vi "SysTime.vi"(5 "Function":enum16{"get_time", "set_time"}(ring), 6 "error in (no error)":errorcluster, 9 "SYSTEMTIME in":T1) -> (0 "error out":errorcluster, 3 "SYSTEMTIME out":T1)   [LabVIEW 2011]
doc: "This VI acts as a Win32 System Call wrapper. Embedded within the VI are \"Call Library\" functions which call various functions from the KERNEL32, GDI, and USER dynamically linked libraries (.DLL's) found in the Windows\\System directory.\n\nThe input is an Enumerated U16 which describes the type of system call to make, and which of the VI's input/output terminals to utilize. A generic \"error?\" boolean is output to indicate any errors with the function calls.\n\nList of Functions and Input/Output Terminals:\n---------------------------------------------------------------------------------------------------------------\n0) get_time: uses the \"SYSTEMTIME out\" terminal only. This call retrieves the system time according to the CPU and operating system. The output is a cluster of eight U16's (the same as the Win32 API description of the SYSTEMTIME structure).\n\n1) set_time: uses both the \"SYSTEMTIME\" and \"SYSTEMTIME out\" terminals. This call will set the system clock to the time and date indicated in the input structure (cluster)."
uses:
  KERNEL32.DLL
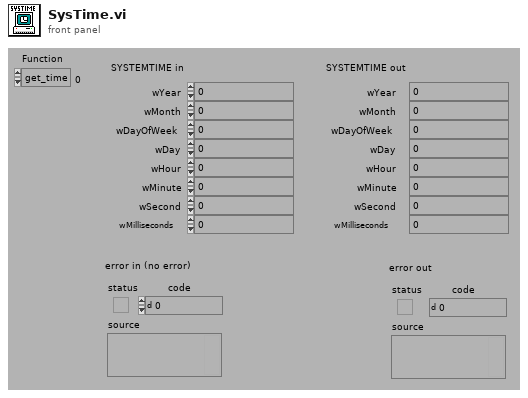
[diagram p1: front panel]
types:
  T1 = cluster{"wYear":u16, "wMonth":u16, "wDayOfWeek":u16, "wDay":u16, "wHour":u16, "wMinute":u16, "wSecond":u16, "wMilliseconds":u16}
  T2 = cluster{"SysTimeStruct[0]":u16, "SysTimeStruct[1]":u16, "SysTimeStruct[2]":u16, "SysTimeStruct[3]":u16, "SysTimeStruct[4]":u16, "SysTimeStruct[5]":u16, "SysTimeStruct[6]":u16, "SysTimeStruct[7]":u16}
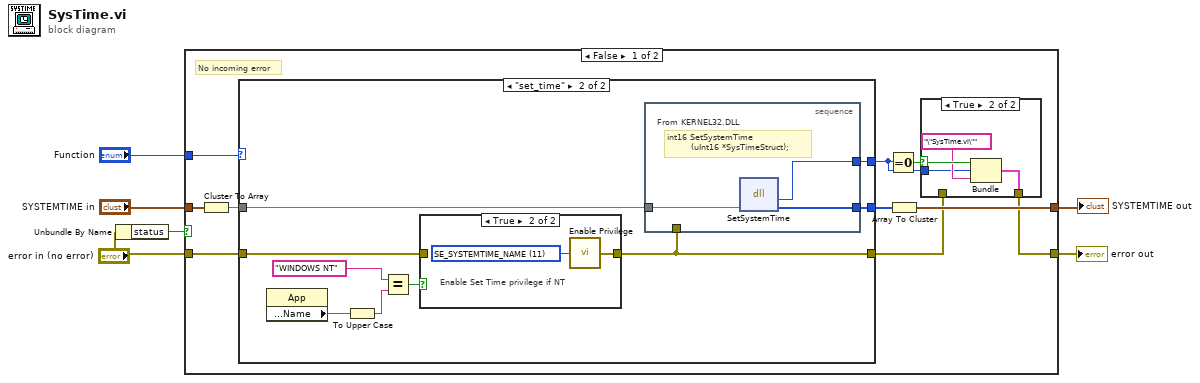
[diagram p0: block diagram]
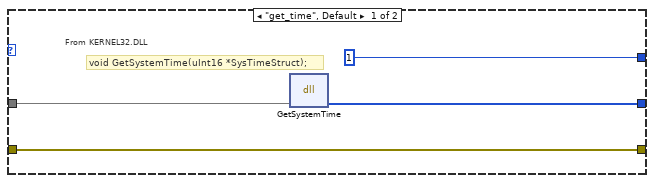
[diagram p3: hidden frame]
diagram:
  n1 = Unbundle By Name("error in (no error)") -> ("status"=w3:bool)
  n2 = case shown="False" w3 {
    tunnel: "SYSTEMTIME in" -> [w16 w41]
    tunnel: [w15 w41] -> w5
    tunnel: "Function" -> [w12 _]
    tunnel: [w10 w42] -> w1
    tunnel: "error in (no error)" -> [w8 w42]
    frame False {
      # "No incoming error"
      n3 = Cluster To Array(cluster=w16) -> (array=w13:u16[])
      n4 = case shown="\"set_time\"" w12 {
        tunnel: [w25 w33] -> w14
        tunnel: w13 -> [w24 w34]
        tunnel: [i16 1 w32] -> w9
        tunnel: w8 -> [w22 w27]
        tunnel: [w22 w26] -> w7
        frame "get_time", Default {
          # "void GetSystemTime(uInt16 *SysTimeStruct);"
          # "From KERNEL32.DLL"
          n5 = dll-call lib="KERNEL32.DLL" fn="GetSystemTime"("SysTimeStruct"=w24) -> ("SysTimeStruct"=w25:u16[])  [unwired: 4 in, 2 out]
        }
        frame "set_time" {
          n6 = property class="App"() -> ("Operating System:Name"=w29:string)  [unwired: 2 in, 2 out]
          n7 = To Upper Case(1:w29) -> (0:w31:string)
          n8 = Equal?(x="WINDOWS NT", y=w31) -> (x = y?=w28:bool)
          n9 = case shown="True" w28 {
            tunnel: w27 -> [w38 _]
            tunnel: [w38 w39] -> w26
            frame False {
            }
            frame True {
              w40 = 11 items=["SE_CREATE_TOKEN_NAME", "SE_ASSIGNPRIMARYTOKEN_NAME", "SE_LOCK_MEMORY_NAME", "SE_INCREASE_QUOTA_NAME", "SE_UNSOLICITED_INPUT_NAME", "SE_MACHINE_ACCOUNT_NAME", "SE_TCB_NAME", "SE_SECURITY_NAME", "SE_TAKE_OWNERSHIP_NAME", "SE_LOAD_DRIVER_NAME", "SE_SYSTEM_PROFILE_NAME", "SE_SYSTEMTIME_NAME", "SE_PROF_SINGLE_PROCESS_NAME", "SE_INC_BASE_PRIORITY_NAME", "SE_CREATE_PAGEFILE_NAME", "SE_CREATE_PERMANENT_NAME", "SE_BACKUP_NAME", "SE_RESTORE_NAME", "SE_SHUTDOWN_NAME", "SE_DEBUG_NAME", "SE_AUDIT_NAME", "SE_SYSTEM_ENVIRONMENT_NAME", "SE_CHANGE_NOTIFY_NAME", "SE_REMOTE_SHUTDOWN_NAME"] ("Privilege (SE_CREATE_TOKEN_NAME)")
              # "Enable Set Time privilege if NT"
              n10 = call "Enable Privilege.vi"("Privilege (SE_CREATE_TOKEN_NAME)"=w40) -> ("error out"=w39:errorcluster)
            }
          }
          n11 = stacked-sequence {
            tunnel: w34 -> [w37]
            tunnel: [w36] -> w33
            tunnel: [w35] -> w32
            tunnel: w26 -> [_]
            frame #0 {
              # "From KERNEL32.DLL"
              # "int16 SetSystemTime\n        (uInt16 *SysTimeStruct);"
              n12 = dll-call lib="KERNEL32.DLL" fn="SetSystemTime"("SysTimeStruct"=w37) -> (w35:i16, "SysTimeStruct"=w36:u16[])  [unwired: 3 in, 2 out]
            }
          }
        }
      }
      n13 = Equal To 0?(x=w9) -> (x = 0?=w11:bool)
      n14 = Array To Cluster(array=w14) -> (cluster=w15:T2)
      n15 = case shown="True" w11 {
        selector: w11 -> [_ w21]
        tunnel: w7 -> [w17 _]
        tunnel: [w17 w19] -> w10
        tunnel: w9 -> [_ w18]
        frame False {
          # "No error"
        }
        frame True {
          n16 = Bundle(w21, w18, "\"SysTime.vi\"") -> (w19:cluster{bool, i16, string})  [unwired: 1 in]
        }
      }
    }
    frame True {
      # "Incoming error"
    }
  }
  "SYSTEMTIME out" <- w5
  "error out" <- w1
